vi "Process data.vi"(8 "error in (no error)":errorcluster, 10 "input array":dbl[][](array[numeric]), 11 "ExampleClassDEdge in":refnum<class "ExampleClassDEdge.lvclass">) -> (0 "error out":errorcluster, 2 "output array":dbl[][](array[numeric]), 3 "ExampleClassDEdge out":refnum<class "ExampleClassDEdge.lvclass">)   [LabVIEW 2012, in "ExampleClassDEdge.lvclass"]
uses:
  ExampleClassDEdge.lvclass
  <vilib>/Analysis/2dsp.llb/2D Convolution (DBL).vi
  <vilib>/Analysis/NI_AALPro.lvlib
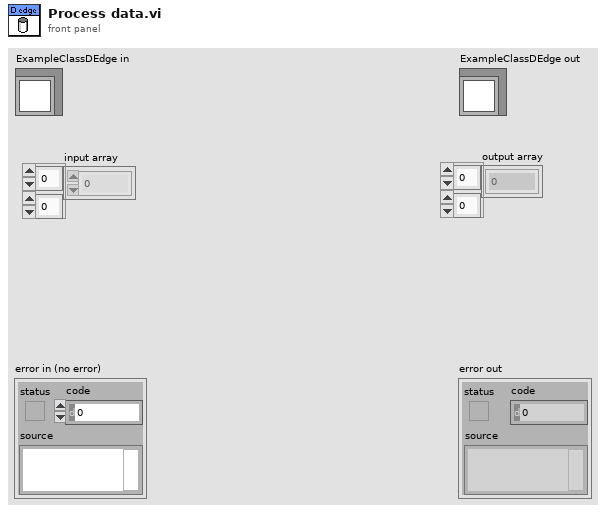
[diagram p1: front panel]
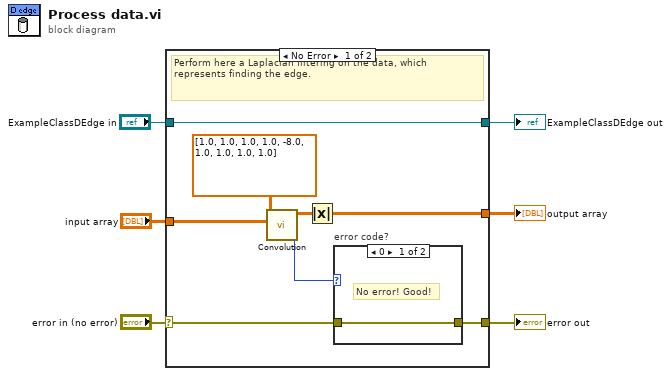
[diagram p0: block diagram]
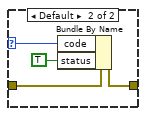
[diagram p2: hidden frame]
diagram:
  n1 = case shown="No Error" "error in (no error)" {
    selector: "error in (no error)" -> [w8 w20]
    tunnel: "input array" -> [w13 w21]
    tunnel: [w11 w21] -> w5
    tunnel: [w9 w20] -> w4
    tunnel: [w7 w22] -> w2
    tunnel: "ExampleClassDEdge in" -> [w7 w22]
    frame No Error {
      # "Perform here a Laplacian filtering on the data, which represents finding the edge."
      n2 = call-poly <vilib>:"Convolution.vi"("Y"=w13, "X"=dbl[][] [[1.0, 1.0, 1.0], [1.0, -8.0, 1.0], [1.0, 1.0, 1.0]]) -> ("error"=w10:i32, "X * Y"=w14:dbl[][])  [unwired: 8 in]
      n3 = Absolute Value(x=w14) -> (abs(x)=w11:dbl[][])
      n4 = case "error code?" shown="0" w10 {
        selector: w10 -> [_ w17]
        tunnel: [w15 w18] -> w9
        tunnel: w8 -> [w15 w19]
        frame 0 {
          # "No error! Good!"
        }
        frame Default {
          n5 = Bundle By Name(cluster=w19, "code"=w17, "status"=TRUE) -> (w18:errorcluster)
        }
      }
    }
    frame Error {
    }
  }
  "error out" <- w4
  "ExampleClassDEdge out" <- w2
  "output array" <- w5
